vi "lecture2-Dataflow Programming.vi"() -> ()   [LabVIEW 2014]
panel:
  out "Result 2":dbl
  out "Result 1":dbl
  in  "Numeric 4":dbl
  in  "Numeric 3":dbl
  in  "Numeric 2":dbl
  in  "Numeric":dbl
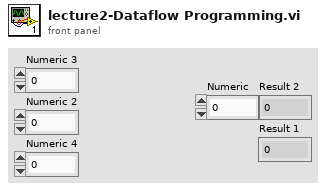
[diagram p1: front panel]
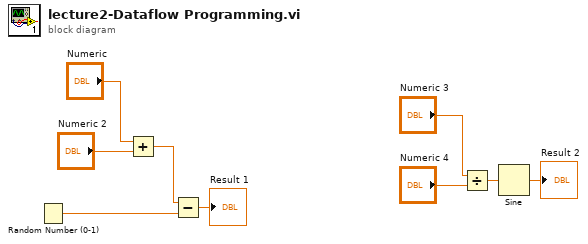
[diagram p0: block diagram]
diagram:
  n1 = Random Number (0-1)() -> (number: 0 to 1=w5:dbl)
  n2 = Add(x="Numeric", y="Numeric 2") -> (x+y=w6:dbl)
  n3 = Subtract(x=w6, y=w5) -> (x-y=→"Result 1":dbl)
  n4 = Divide(x="Numeric 3", y="Numeric 4") -> (x/y=w3:dbl)
  n5 = Sine(x=w3) -> (sin(x)=→"Result 2":dbl)
